vi "Custom source-meter - IV sweep.vi"(4 "XY Graph to update":refnum<vi>, 6 "Status string reference":refnum<vi>, 8 "Error In":errorcluster, 9 "Stop occurrence":refnum<k4>, 10 "IV properties":T1={"T"=0.0, "Vstart"=-0.5, "Vstop"=0.5, "Vpoints"=10.0, "Settling"=0.01, "I limit"=0.1, "Log mapping"=FALSE, "Averaging"=0.0}, 11 "Source-meter":T2) -> (0 "Error Out":errorcluster, 2 "Voltage (V)":dbl[](array[numeric]), 3 "Current (A)":dbl[](array[numeric]))   [LabVIEW 2019]
doc: "This subVI is meant to perform a I-V sweep (including data acquisition). Sweep parameters and your custom settings are made available to you. Remebmer to return measured data to current and voltage arrays."
uses:
  Type defs/Source-meter Type Def.ctl
  Custom source-meter settings.ctl
  Type defs/IV properties Type Def.ctl
panel:
  # "Place all operations necessary to perform IV sweep in this VI"
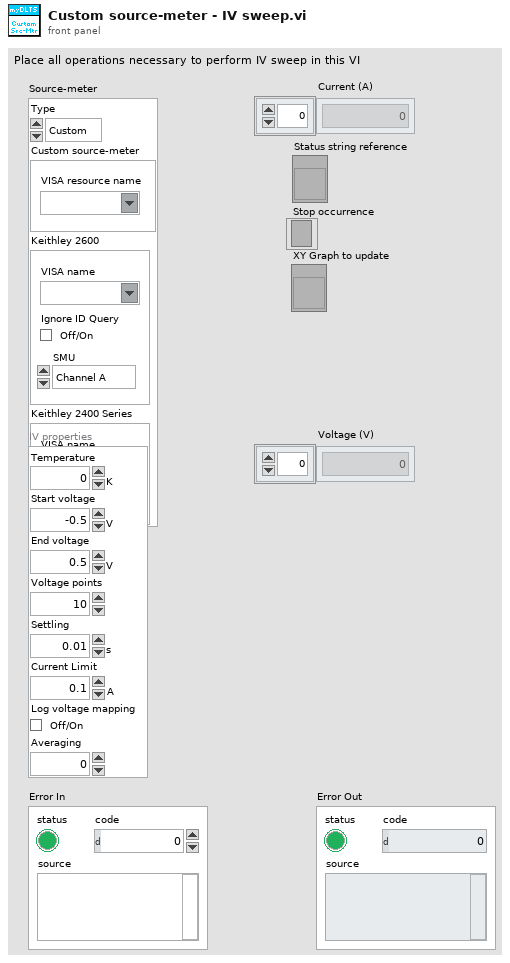
[diagram p1: front panel]
types:
  T1 = typedef "IV properties Type Def.ctl" = cluster{"T":dbl[unit], "Vstart":dbl[unit], "Vstop":dbl[unit], "Vpoints":dbl, "Settling":dbl[unit], "I limit":dbl[unit], "Log mapping":bool, "Averaging":dbl}
  T2 = typedef "Source-meter Type Def.ctl" = cluster{"Type":enum16{"Custom", "Keithley 2600 Series", "Keithley 2400 Series"}, "Custom source-meter":T3, "Keithley 2600":cluster{"VISA name":refnum<visa-resource-name>, "Ignore ID Query":bool, "SMU":enum16{"Channel A", "Channel B"}}, "Keithley 2400 Series":cluster{"VISA name":refnum<visa-resource-name>, "Ignore ID Query":bool}}
  T3 = typedef "Custom source-meter settings.ctl" = cluster{"VISA resource name":refnum<visa-resource-name>}
  T4 = cluster{"Voltage points":dbl[], "Current points":dbl[]}
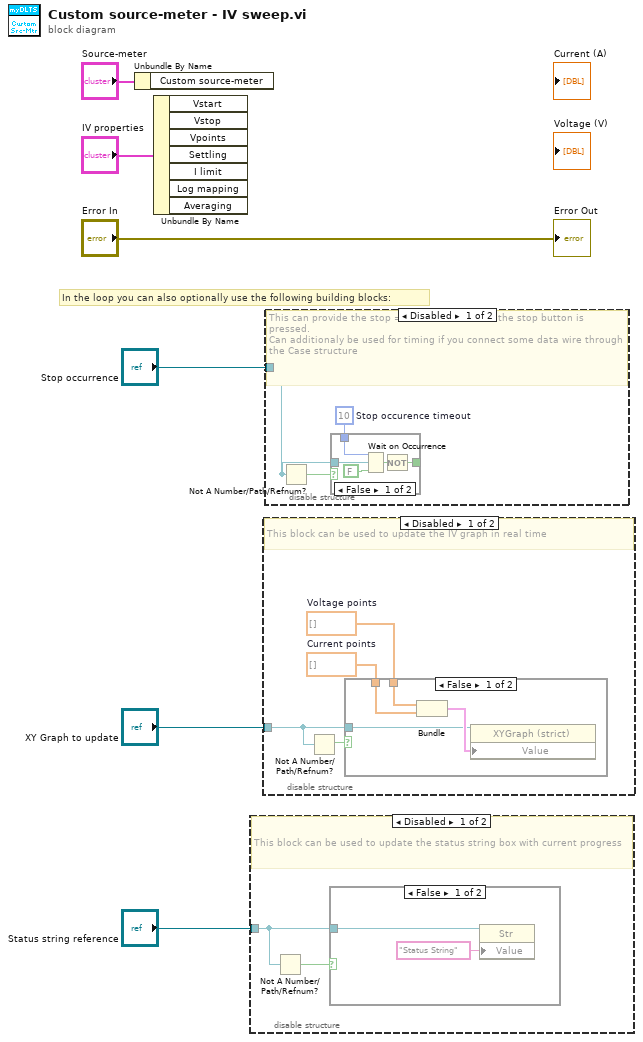
[diagram p0: block diagram]
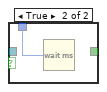
[diagram p6: hidden frame]
diagram:
  # "In the loop you can also optionally use the following building blocks:"
  n1 = Unbundle By Name("Source-meter") -> ()  [unwired: 1 out]
  n2 = Unbundle By Name("IV properties") -> ()  [unwired: 7 out]
  n3 = disable-structure shown="Disabled" {
    disable-tunnel: "Status string reference" -> [w7 _]
    frame Disabled {
      # "This block can be used to update the status string box with current progress"
      n4 = Not A Number/Path/Refnum?(number/path/refnum=w7) -> (NaN/Path/Refnum?=w8:bool)
      n5 = case shown="False" w8 {
        tunnel: w7 -> [w9 _]
        frame False {
          n6 = property class="Str"(reference=w9, "Value"="Status String") -> ()  [unwired: 1 in, 2 out]
        }
        frame True {
        }
      }
    }
    frame Enabled {
    }
  }
  n7 = disable-structure shown="Disabled" {
    disable-tunnel: "XY Graph to update" -> [w14 _]
    frame Disabled {
      w11 = dbl[] []  # Current points
      w12 = dbl[] []  # Voltage points
      # "This block can be used to update the IV graph in real time"
      n8 = Not A Number/Path/Refnum?(number/path/refnum=w14) -> (NaN/Path/Refnum?=w13:bool)
      n9 = case shown="False" w13 {
        tunnel: w11 -> [w18 _]
        tunnel: w14 -> [w16 _]
        tunnel: w12 -> [w15 _]
        frame False {
          n10 = Bundle("Voltage points"=w15, "Current points"=w18) -> (w17:T4)  [unwired: 1 in]
          n11 = property on="Property Node" class="XYGraph (strict)"(reference=w16, "Value"=w17) -> ()  [unwired: 1 in, 2 out]
        }
        frame True {
        }
      }
    }
    frame Enabled {
    }
  }
  n12 = disable-structure shown="Disabled" {
    disable-tunnel: "Stop occurrence" -> [w20 _]
    frame Disabled {
      w19 = u32 10  # Stop occurence timeout
      # "This can provide the stop = true boolean when the stop button is pressed.\nCan additionaly be used for timing if you connect some data wire through the Case structure"
      n13 = Not A Number/Path/Refnum?(number/path/refnum=w20) -> (NaN/Path/Refnum?=w21:bool)
      n14 = case shown="False" w21 {
        tunnel: [w25 _] -> _
        tunnel: w19 -> [w24 w27]
        tunnel: w20 -> [w23 _]
        frame False {
          n15 = Wait on Occurrence(1:FALSE ("ignore previous (T)"), 2:w23, 3:w24) -> (0:w26:bool)
          n16 = Not(x=w26) -> (.not. x?=w25:bool)
        }
        frame True {
          n17 = Wait (ms)(milliseconds to wait=w27) -> ()  [unwired: 1 out]
        }
      }
    }
    frame Enabled {
    }
  }
  "Error Out" <- "Error In"
